vi "ITX to LV 2.1.vi"(8 "error in":errorcluster, 11 "file (use dialog)":path=path "P:/sample/GaAs/GaAs quantum dots/2008/PL Map/A1 735/060731ASBA_A1_6.0.itx") -> (0 "error out":errorcluster, 1 "1D arrays":dbl[][](array[numeric]), 2 "2D array":dbl[][](array[numeric]), 3 "Data (Dictionary)":cluster{"key":variant, "value":variant}[](array[cluster]), 4 "Notes":string, 5 "wave names":string[](array[string]), 6 "Commands":string)   [LabVIEW 2016, in "LVtoITX.lvclass"]
uses:
  LVtoITX.lvclass
panel:
  out "base wavenames":string[](array[string])
  out "parse 2 (ms)":u32
  out "parse 2":u32
  out "parse 1 (ms)":u32
  out "open file (ms)":u32
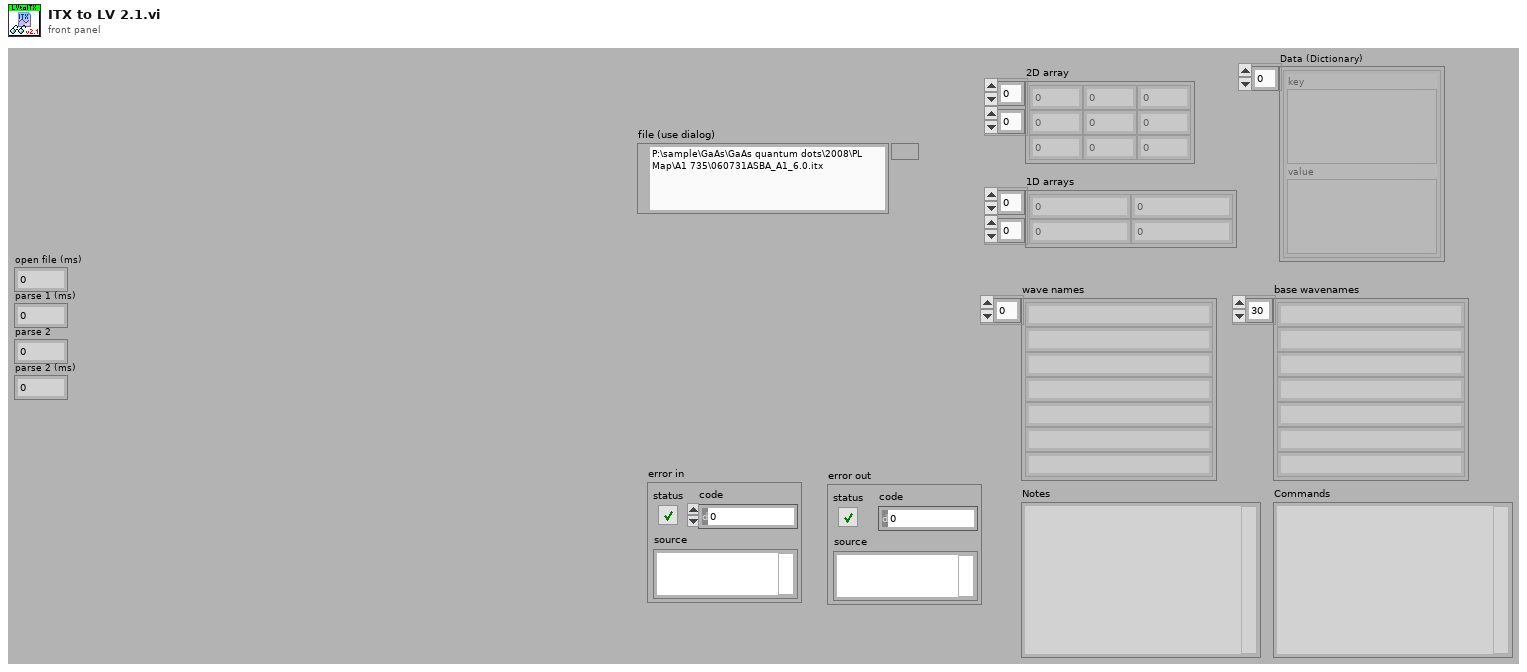
[diagram p1: front panel]
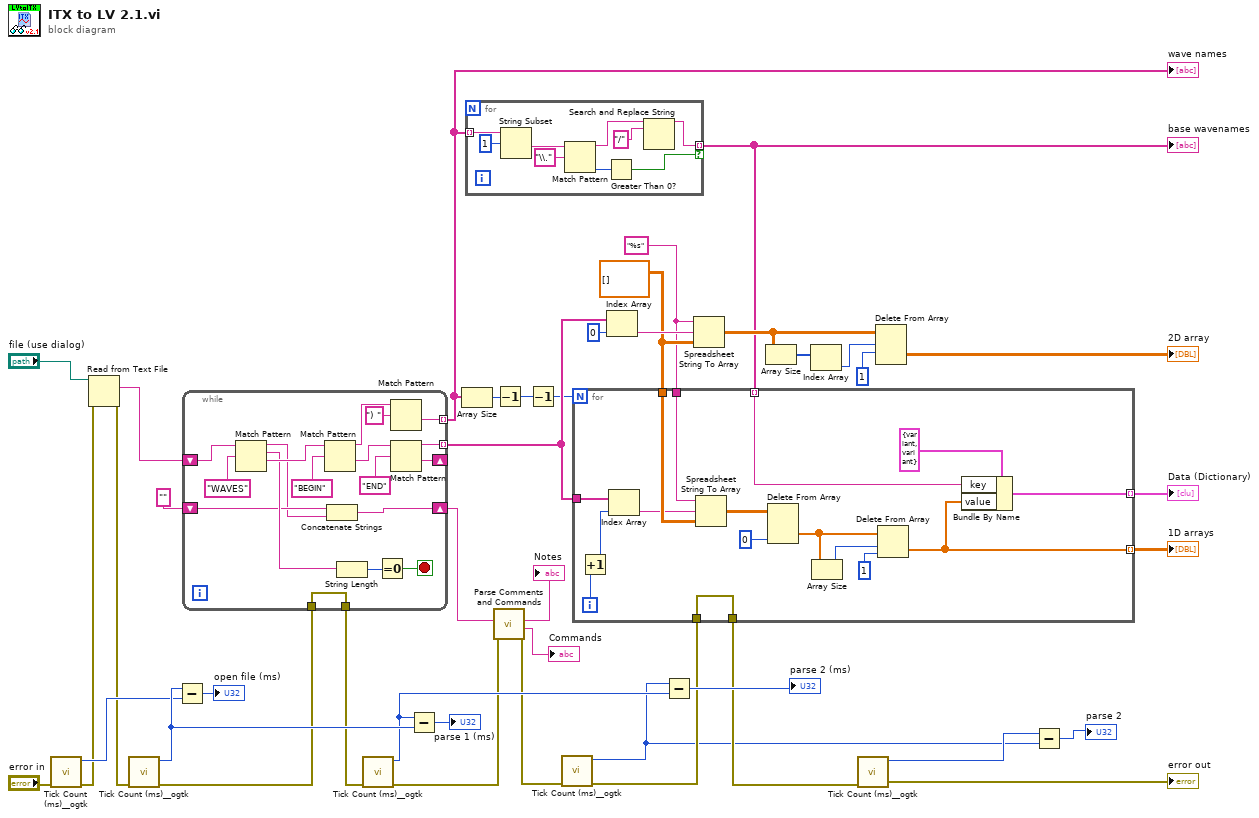
[diagram p0: block diagram]
diagram:
  w33 = "%s" ("format string")
  w35 = dbl[][] [] ("array type (2D Dbl)")
  n1 = call <userlib>:"Tick Count (ms)__ogtk.vi"("error in (no error)"="error in") -> ("error out"=w22:errorcluster, "millisecond timer value"=w24:u32)  [unwired: 9 in]
  n2 = Read from Text File(file (use dialog)="file (use dialog)", error in=w22) -> (text=w3:string, error out=w21:errorcluster)  [unwired: 1 in, 3 out]
  n3 = call <userlib>:"Tick Count (ms)__ogtk.vi"("error in (no error)"=w21) -> ("error out"=w19:errorcluster, "millisecond timer value"=w27:u32)  [unwired: 9 in]
  n4 = Subtract(x=w27, y=w24) -> (x-y=→"open file (ms)":u32)
  n5 = while {
    tunnel: [w57] -> w34 mode=indexing
    shift-right: [w58] -> _
    shift-left: w3 -> [w45]
    tunnel: [w53] -> w13 mode=indexing
    shift-right: [w48] -> w18
    shift-left: "" ("regular expression") -> [w47]
    tunnel: [w43] -> w20
    tunnel: w19 -> [w43]
    stop <- w54 stop-if-true
    n6 = Match Pattern(string=w45, regular expression="WAVES") -> (before substring=w46:string, match substring=w56:string, after substring=w60:string)  [unwired: 2 out]
    n7 = Match Pattern(string=w60, regular expression="BEGIN" ("regular expression 2")) -> (before substring=w44:string, after substring=w59:string)  [unwired: 3 out]
    n8 = Concatenate Strings(w47, w46) -> (w48:string)
    n9 = String Length(string=w56) -> (length=w55:i32)
    n10 = Equal To 0?(x=w55) -> (x = 0?=w54:bool)
    n11 = Match Pattern(string=w44, regular expression=") ") -> (after substring=w53:string)  [unwired: 4 out]
    n12 = Match Pattern(string=w59, regular expression="END" ("regular expression 3")) -> (before substring=w57:string, after substring=w58:string)  [unwired: 3 out]
  }
  "wave names" <- w13
  n13 = call <userlib>:"Tick Count (ms)__ogtk.vi"("error in (no error)"=w20) -> ("error out"=w15:errorcluster, "millisecond timer value"=w25:u32)  [unwired: 9 in]
  n14 = Subtract(x=w25, y=w27) -> (x-y=→"parse 1 (ms)":u32)
  n15 = Array Size(array=w13) -> (size(s)=w14:i32)
  n16 = for {
    tunnel: w13 -> [w68] mode=indexing
    tunnel: [w61] -> w2 mode=indexing if=w64
    n17 = String Subset(string=w68, offset (0)=1) -> (substring=w67:string)  [unwired: 1 in]
    n18 = Match Pattern(string=w67, regular expression="\\.") -> (before substring=w62:string, offset past match=w65:i32)  [unwired: 1 in, 2 out]
    n19 = Greater Than 0?(x=w65) -> (x > 0?=w64:bool)
    n20 = Search and Replace String(input string=w62, search string="/") -> (result string=w61:string)  [unwired: 6 in, 3 out]
  }
  "base wavenames" <- w2
  n21 = call "Parse Comments and Commands.vi"("error in"=w15, "Igor Comments and Commands"=w18) -> ("error out"=w11:errorcluster, "Commands"=→"Commands":string, "Comments"=→"Notes":string)  [unwired: 7 in]
  n22 = Decrement(x=w14) -> (x-1=w32:i32)
  n23 = Decrement(x=w32) -> (x-1=w31:i32)
  n24 = call <userlib>:"Tick Count (ms)__ogtk.vi"("error in (no error)"=w11) -> ("error out"=w10:errorcluster, "millisecond timer value"=w6:u32)  [unwired: 9 in]
  n25 = for {
    N: w31 -> [_]
    tunnel: [w72] -> w30 mode=indexing
    tunnel: w35 -> [w80]
    tunnel: w34 -> [w79]
    tunnel: w33 -> [w78]
    tunnel: w10 -> [w74]
    tunnel: [w74] -> w9
    tunnel: w2 -> [w71] mode=indexing
    tunnel: [w70] -> w1 mode=indexing
    i -> [w77]
    n26 = Increment(x=w77) -> (x+1=w76:i32)
    n27 = Index Array(array=w79, index=w76) -> (element=w75:string)
    n28 = Spreadsheet String To Array(format string=w78, spreadsheet string=w75, array type (2D Dbl)=w80) -> (array=w84:dbl[][])  [unwired: 1 out]
    n29 = Delete From Array(array=w84, index (col)=0 ("disabled index (col)")) -> (deleted portion=w83:dbl[])  [unwired: 2 in, 1 out]
    n30 = Array Size(array=w83) -> (size(s)=w82:i32)
    n31 = Delete From Array(array=w83, length=w82, index=1) -> (deleted portion=w72:dbl[])  [unwired: 1 out]
    n32 = Bundle By Name(cluster=cluster{"key":variant, "value":variant} {"key"=variant, "value"=variant} ("key-value"), "key"=w71, "value"=w72) -> (w70:cluster{"key":variant, "value":variant})
  }
  "1D arrays" <- w30
  "Data (Dictionary)" <- w1
  n33 = Index Array(array=w34, index=0) -> (element=w41:string)
  n34 = Subtract(x=w6, y=w25) -> (x-y=→"parse 2 (ms)":u32)
  n35 = Spreadsheet String To Array(format string=w33, spreadsheet string=w41, array type (2D Dbl)=w35) -> (array=w39:dbl[][])  [unwired: 1 out]
  n36 = Array Size(array=w39) -> (size(s)=w38:i32[])
  n37 = Index Array(array=w38) -> (element=w36:i32)  [unwired: 1 in]
  n38 = call <userlib>:"Tick Count (ms)__ogtk.vi"("error in (no error)"=w9) -> ("error out"=→"error out":errorcluster, "millisecond timer value"=w8:u32)  [unwired: 9 in]
  n39 = Delete From Array(array=w39, length=w36, index (row)=1) -> (deleted portion=→"2D array":dbl[][])  [unwired: 1 in, 1 out]
  n40 = Subtract(x=w8, y=w6) -> (x-y=→"parse 2":u32)
